vi "Double Definition.vi"(11 "Double in":refnum<class "Double.lvclass">) -> (2 "Definition":T1)   [LabVIEW 2020, in "Conditum.lvlib" / "Columns.lvlib" / "Double.lvclass"]
uses:
  Double.lvclass
  Double.lvclass/Double.ctl
  Definition.ctl
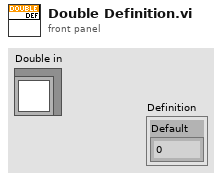
[diagram p1: front panel]
types:
  T1 = typedef "Conditum.lvlib/Columns.lvlib/Double.lvclass/Definition.ctl" = cluster{"Default":dbl}
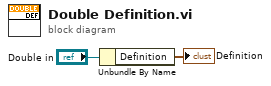
[diagram p0: block diagram]
diagram:
  n1 = Unbundle By Name("Double in") -> ("Definition"=→"Definition":T1)
